vi "CM-Show AOAI Connections.vi"(0 "slot ctl refs":refnum<vi>[](array[refnum]), 5 "Tables By Device":T1(array[cluster]), 7 "Endpoints":cluster{"Name":string[]}[](array[cluster]), 11 "error in (no error)":errorcluster) -> (4 "slot ctl refs out":refnum<vi>[](array[refnum]), 15 "error out":errorcluster)   [LabVIEW 2020]
uses:
  Type Defs/General PXISlot XControl/PXISlotGP.xctl
panel:
  out "Numeric":i32
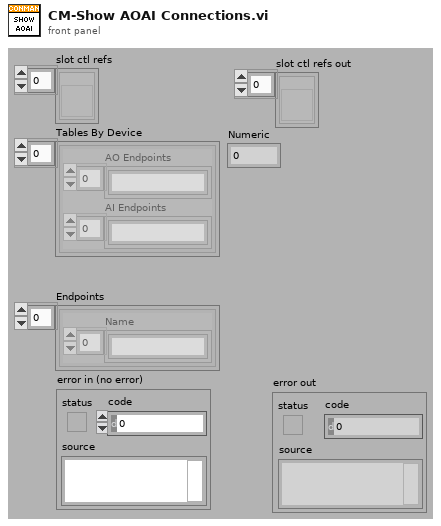
[diagram p1: front panel]
types:
  T1 = cluster{"AO Endpoints":string[], "AI Endpoints":string[]}[]
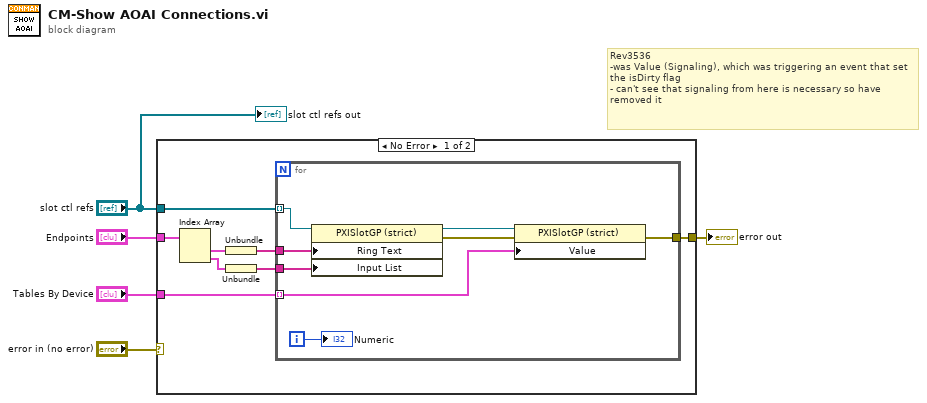
[diagram p0: block diagram]
diagram:
  # "Rev3536\n-was Value (Signaling), which was triggering an event that set the isDirty flag\n- can't see that signaling from here is necessary so have removed it"
  n1 = case shown="No Error" "error in (no error)" {
    selector: "error in (no error)" -> [_ w22]
    tunnel: "slot ctl refs" -> [w13 _]
    tunnel: "Tables By Device" -> [w12 _]
    tunnel: "Endpoints" -> [w11 _]
    tunnel: [w6 w22] -> w2
    frame No Error {
      n2 = Index Array(array=w11) -> (element #1=w10:cluster{"Name":string[]}, element #2=w8:cluster{"Name":string[]})  [unwired: 2 in]
      n3 = Unbundle(w10) -> ("Name"=w9:string[])
      n4 = Unbundle(w8) -> ("Name"=w7:string[])
      n5 = for {
        tunnel: w13 -> [w19] mode=indexing
        tunnel: w12 -> [w21] mode=indexing
        tunnel: w9 -> [w18]
        tunnel: w7 -> [w17]
        tunnel: [w15] -> w6
        i -> [w14]
        n6 = property class="PXISlotGP (strict)"(reference=w19, "Ring Text"=w18, "Input List"=w17) -> (reference out=w20:refnum<vi>, error out=w16:errorcluster)  [unwired: 1 in]
        n7 = property class="PXISlotGP (strict)"(reference=w20, error in=w16, "Value"=w21) -> (error out=w15:errorcluster)  [unwired: 1 out]
        "Numeric" <- w14
      }
    }
    frame Error {
    }
  }
  "error out" <- w2
  "slot ctl refs out" <- "slot ctl refs"
